vi "Auto_Match.vi"() -> ()   [LabVIEW 2015]
panel:
  out "Number of Iterations":i32
  out "Current Number":u32 format="%#.0f"
  in  "Number to Match":u32 max=1000 step=1
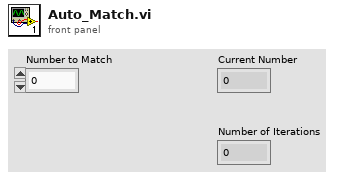
[diagram p1: front panel]
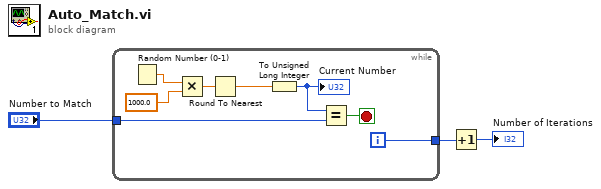
[diagram p0: block diagram]
diagram:
  n1 = while {
    tunnel: "Number to Match" -> [w6]
    tunnel: [w9] -> w2
    i -> [w9]
    stop <- w4 stop-if-true
    n2 = Random Number (0-1)() -> (number: 0 to 1=w11:dbl)
    n3 = Multiply(x=w11, y=1000.0) -> (x*y=w8:dbl)
    n4 = Round To Nearest(number=w8) -> (nearest integer value=w7:dbl)
    n5 = To Unsigned Long Integer(number=w7) -> (unsigned 32bit integer=w5:u32)
    "Current Number" <- w5
    n6 = Equal?(x=w5, y=w6) -> (x = y?=w4:bool)
  }
  n7 = Increment(x=w2) -> (x+1=→"Number of Iterations":i32)
